vi "PicoScope3000aAWG.vi"(6 "Arbitrary Waveform Settings":T2 {"Index Mode" items=["Single", "Dual", "Quad"]}, 7 "Standard Waveform Settings":T3={"Start Frequency"=1000.0, "Stop Frequency"=1000.0, "Increment"=0.0, "Dwell Time (seconds)"=0.0} {"Stop Frequency" min=0.03 max=1000000.0 format="%#_6p"; "Start Frequency" min=0.03 max=1000000.0 format="%#_6p"}, 8 "Device Info":T1, 9 "General AWG Settings":T4={"Peak-to-Peak Voltage (microvolts)"=2000000, "Offset Voltage (microvolts)"=0, "Wave Type"=0, "Sweep Type"=0, "Shots"=0, "Sweeps"=0, "Trigger Type"=0, "Trigger Source"=0, "Ext. Threshold (ADC count)"=0, "White Noise/PRBS"=0} {"White Noise/PRBS" items=["Normal", "White Noise", "PRBS"]; "Trigger Source" items=["None", "Scope Trigger", "Aux. In", "Ext. In", "Software Trigger"]; "Trigger Type" items=["Rising", "Falling", "Gate High", "Gate Low"]; "Sweep Type" items=["Up", "Down", "Up-Down", "Down-Up"]; "Wave Type" items=["Sine"=0, "Square"=1, "Triangle"=2, "Ramp Up"=3, "Ramp Down"=4, "DC"=8, "Arbitrary"=6]}, 10 "Handle In":i16, 11 "error in":errorcluster) -> (0 "Trigger Source Out":i32, 1 "Arbitrary\nWaveform Graph":i16[](graph), 2 "Handle Out":i16, 3 "error out":errorcluster)   [LabVIEW 2010]
doc: "This VI can be used to control the arbitrary waveform generator. Standard waveforms can be selected or arbitrary waveform can be selected under 'Wave Type'. There are three settings clusters: general settings that apply to both arbitrary and standard waveforms, settings that apply only to standard waveforms and settings that apply only to arbitrary waveforms. It is not necessary to connect all of these clusters if only using arbitrary waveforms or only using standard waveforms are required.\n\nWhen selecting arbitrary waveform, it is necessary to specify a text file containing the wave form. This text file should have a single value on each line in the range -1 to 1. For further information on the settings, see descriptions of ps3000aSetSigGenBuiltIn and ps3000aSetSigGenArbitrary."
uses:
  PS3000a.dll
panel:
  # "Sweep is disabled when 'Increment' or 'Dwell Time' is set to 0, then 'Start frequency' is used"
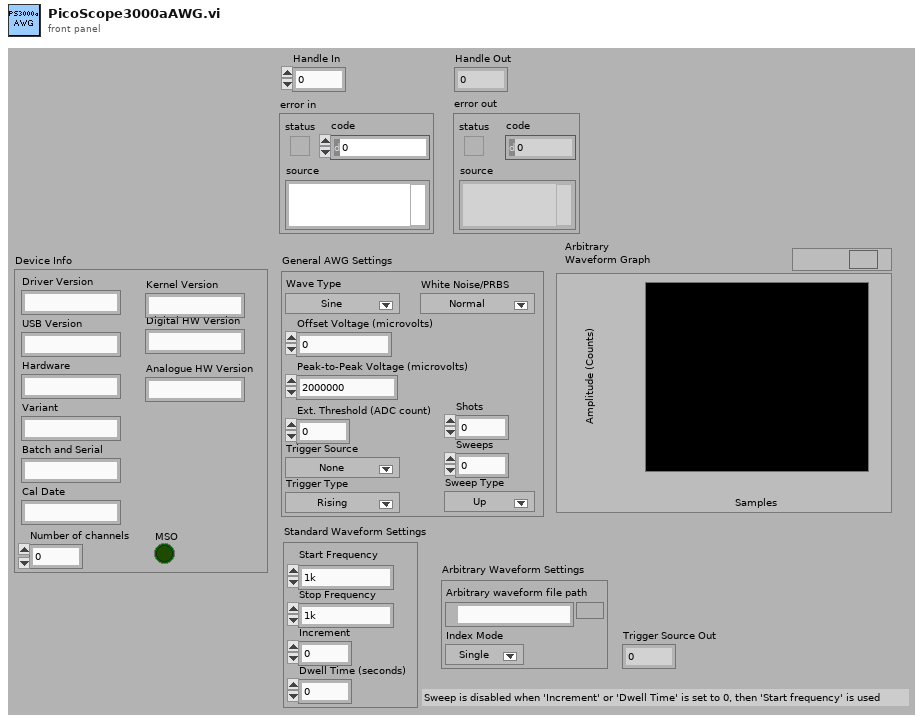
[diagram p1: front panel]
types:
  T1 = cluster{"Driver Version":string, "USB Version":string, "Hardware":string, "Variant":string, "Batch and Serial":string, "Cal Date":string, "Kernel Version":string, "Digital HW Version":string, "Analogue HW Version":string, "MSO":bool, "Number of channels":i16}
  T2 = cluster{"Arbirary waveform file path":path, "Index Mode":u32}
  T3 = cluster{"Start Frequency":dbl, "Stop Frequency":dbl, "Increment":dbl, "Dwell Time (seconds)":dbl}
  T4 = cluster{"Peak-to-Peak Voltage (microvolts)":u32, "Offset Voltage (microvolts)":i32, "Wave Type":i16, "Sweep Type":i32, "Shots":u32, "Sweeps":u32, "Trigger Type":i32, "Trigger Source":i32, "Ext. Threshold (ADC count)":i16, "White Noise/PRBS":u32}
  T5 = cluster{"status":bool, "code":u32, "source":string}
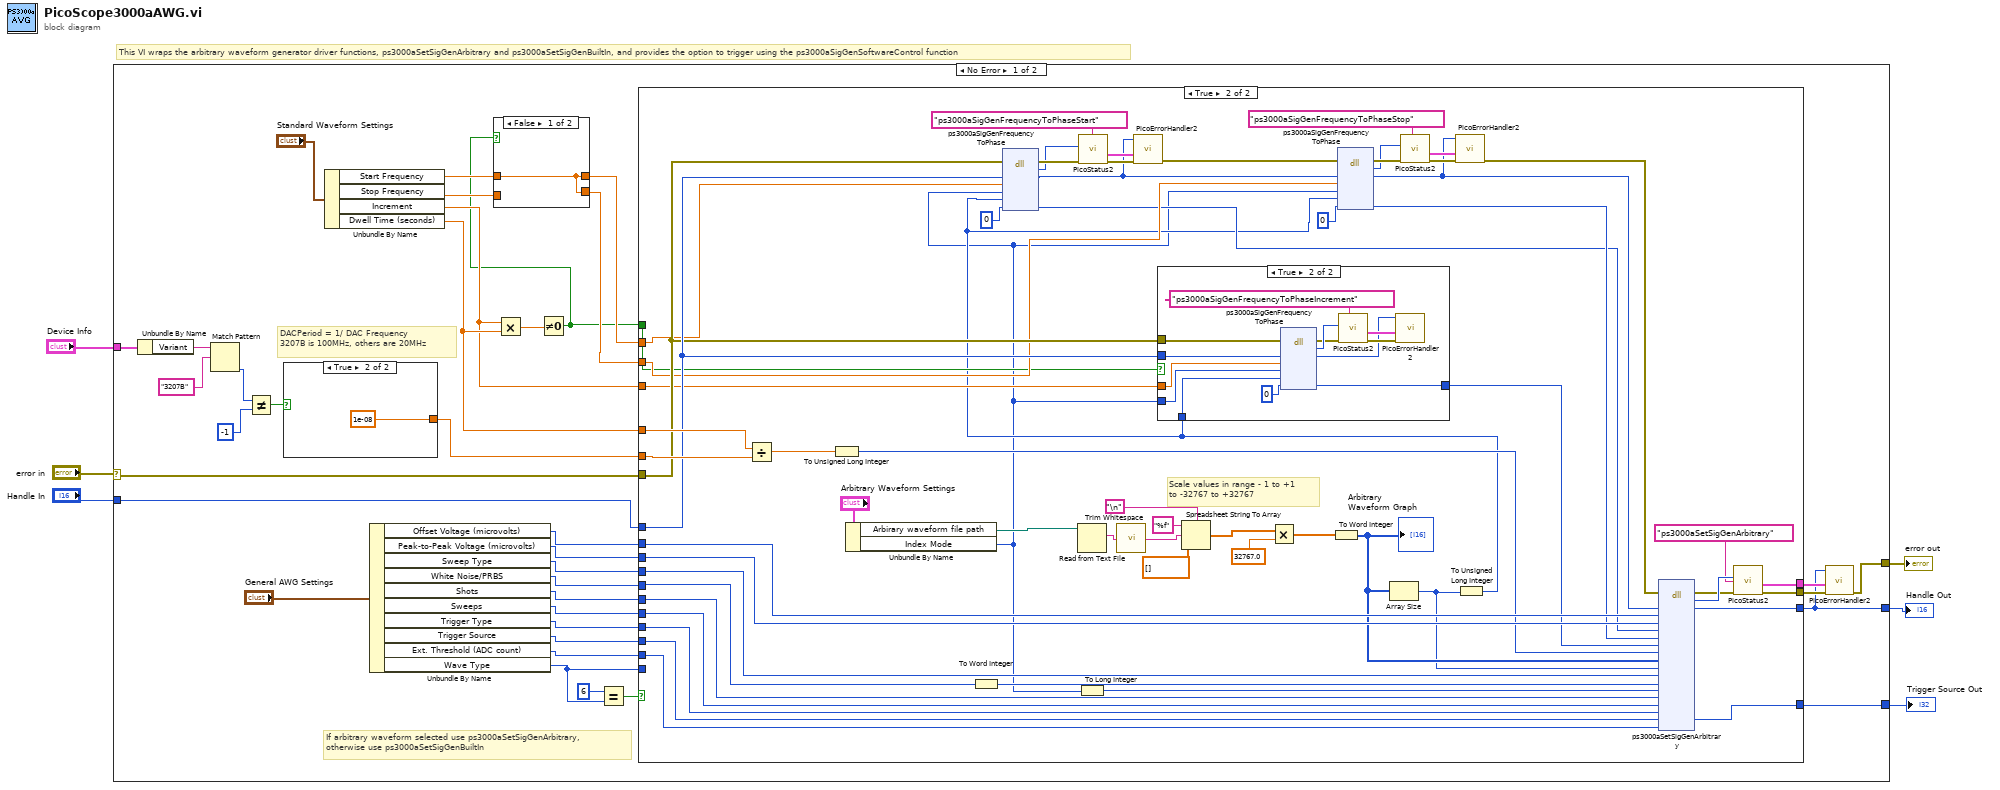
[diagram p0: block diagram]
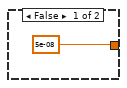
[diagram p2: hidden frame]
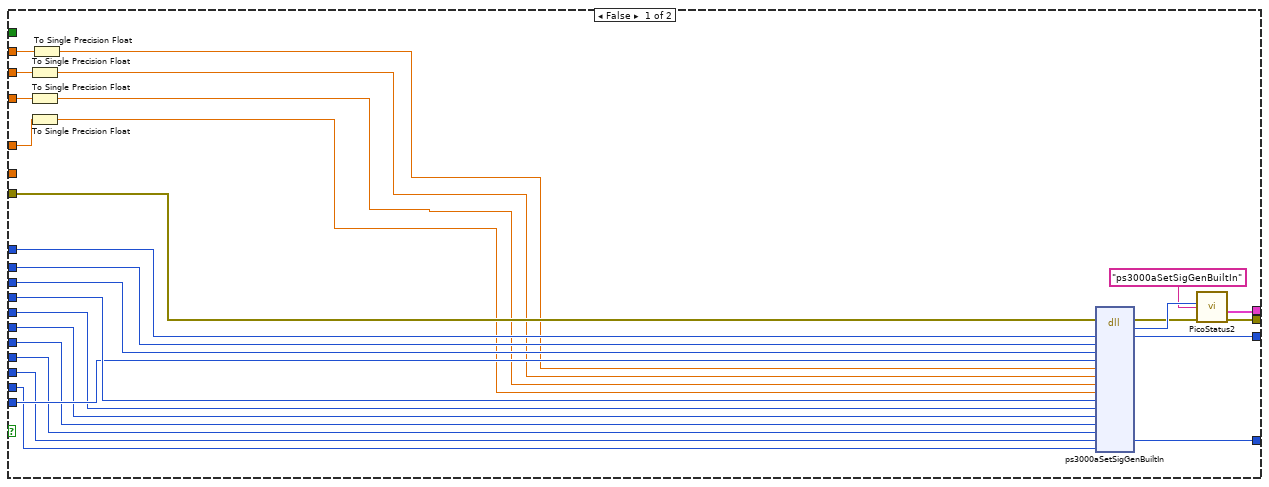
[diagram p4: hidden frame]
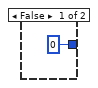
[diagram p5: hidden frame]
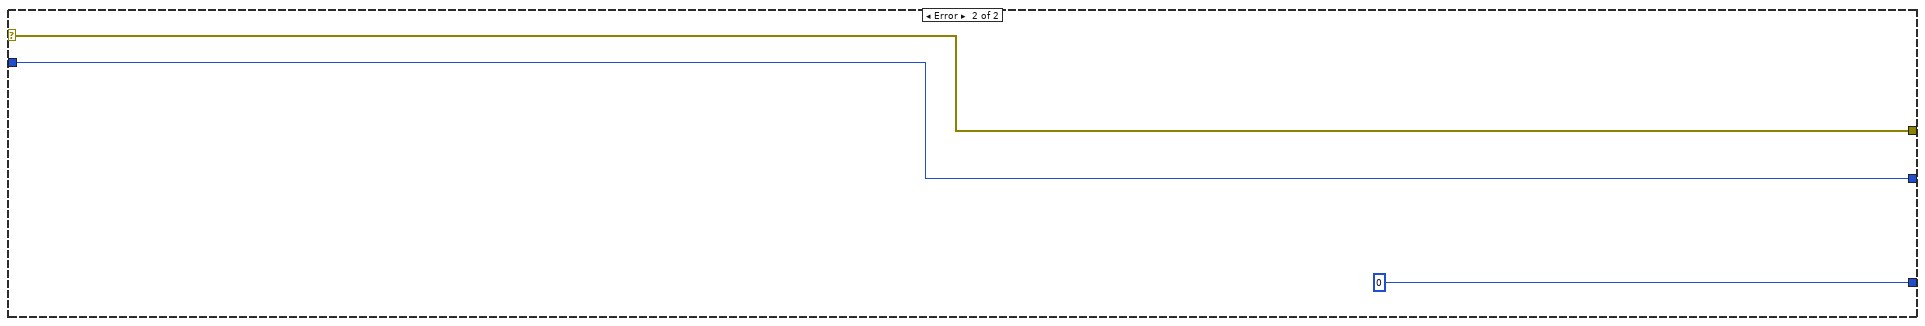
[diagram p6: hidden frame]
diagram:
  # "This VI wraps the arbitrary waveform generator driver functions, ps3000aSetSigGenArbitrary and ps3000aSetSigGenBuiltIn, and provides the option to trigger using the ps3000aSigGenSoftwareControl function"
  n1 = case shown="No Error" "error in" {
    selector: "error in" -> [w27 w152]
    tunnel: [w7 w151] -> w6
    tunnel: "Handle In" -> [w40 w151]
    tunnel: [w39 w152] -> w4
    tunnel: [w25 0] -> w2
    tunnel: "Device Info" -> [w10 _]
    frame No Error {
      # "DACPeriod = 1/ DAC Frequency\n3207B is 100MHz, others are 20MHz"
      # "If arbitrary waveform selected use ps3000aSetSigGenArbitrary, \notherwise use ps3000aSetSigGenBuiltIn"
      n2 = Unbundle By Name(w10) -> ("Variant"=w11:string)
      n3 = Match Pattern(string=w11, regular expression="3207B") -> (offset past match=w12:i32)  [unwired: 1 in, 3 out]
      n4 = Not Equal?(x=w12, y=-1 ("x")) -> (x != y?=w9:bool)
      n5 = case shown="True" w9 {
        tunnel: [5e-08 ("y") 1e-08 ("y")] -> w14
        frame False {
        }
        frame True {
        }
      }
      n6 = Unbundle By Name("Standard Waveform Settings") -> ("Start Frequency"=w23:dbl, "Stop Frequency"=w22:dbl, "Increment"=w19:dbl, "Dwell Time (seconds)"=w20:dbl)
      n7 = Unbundle By Name("General AWG Settings") -> ("Offset Voltage (microvolts)"=w37:i32, "Peak-to-Peak Voltage (microvolts)"=w36:u32, "Sweep Type"=w35:i32, "White Noise/PRBS"=w34:u32, "Shots"=w33:u32, "Sweeps"=w32:u32, "Trigger Type"=w31:i32, "Trigger Source"=w30:i32, "Ext. Threshold (ADC count)"=w29:i16, "Wave Type"=w28:i16)
      n8 = Multiply(x=w19, y=w20) -> (x*y=w21:dbl)
      n9 = Not Equal To 0?(x=w21) -> (x != 0?=w16:bool)
      n10 = case shown="False" w16 {
        tunnel: [w45 w47] -> w18
        tunnel: w22 -> [_ w47]
        tunnel: w23 -> [w45 w46]
        tunnel: [w45 w46] -> w17
        frame False {
        }
        frame True {
        }
      }
      n11 = Equal?(x=i16 6, y=w28) -> (x = y?=w42:bool)
      n12 = case shown="True" w42 {
        tunnel: [w74 w130] -> w7
        tunnel: w40 -> [w73 w96]
        tunnel: [w71 w127] -> w26
        tunnel: w37 -> [w69 w126]
        tunnel: w36 -> [w68 w125]
        tunnel: w35 -> [w67 w124]
        tunnel: w34 -> [w49 w83]
        tunnel: w33 -> [w65 w123]
        tunnel: w32 -> [w64 w122]
        tunnel: w31 -> [w63 w121]
        tunnel: w30 -> [w62 w120]
        tunnel: w29 -> [w61 w119]
        tunnel: w28 -> [w66 _]
        tunnel: [w60 w117] -> w25
        tunnel: w27 -> [w59 w95]
        tunnel: w20 -> [w57 w110]
        tunnel: w19 -> [w56 w92]
        tunnel: w18 -> [w55 w93]
        tunnel: w17 -> [w54 w94]
        tunnel: w14 -> [_ w111]
        tunnel: w16 -> [_ w87]
        tunnel: [w48 w75] -> w8
        frame False {
          n13 = To Single Precision Float(number=w55) -> (single precision float=w51:sgl)
          n14 = To Single Precision Float(number=w56) -> (single precision float=w52:sgl)
          n15 = To Single Precision Float(number=w57) -> (single precision float=w53:sgl)
          n16 = To Single Precision Float(number=w54) -> (single precision float=w50:sgl)
          n17 = dll-call lib="ps3000a.dll" fn="ps3000aSetSigGenBuiltIn" ("ps3000.dll:_ps3000_open_unit@0")(error in=w59, "handle"=w73, "offsetVoltage"=w69, "pkToPk"=w68, "waveType"=w66, "startFrequency"=w50, "stopFrequency"=w51, "increment"=w52, "dwellTime"=w53, "sweepType"=w67, "whiteNoise"=w49, "shots"=w65, "sweeps"=w64, "triggerType"=w63, "triggerSource"=w62, "extInThreshold"=w61) -> (error out=w58:errorcluster, "PICO_STATUS"=w72:u32, "handle"=w74:i16, "triggerSource"=w60:i32)  [unwired: 15 in, 1 out]
          n18 = call "PicoStatus2.vi"("PICO source"="ps3000aSetSigGenBuiltIn" ("source"), "Error in"=w58, "PICO STATUS"=w72) -> ("error out"=w71:errorcluster, "PICO_STATUS out"=w48:T5)  [unwired: 5 in]
        }
        frame True {
          # "Scale values in range - 1 to +1 \nto -32767 to +32767"
          n19 = Divide(x=w110, y=w111) -> (x/y=w112:dbl)
          n20 = To Unsigned Long Integer(number=w112) -> (unsigned 32bit integer=w109:u32)
          n21 = Unbundle By Name("Arbitrary Waveform Settings") -> ("Arbirary waveform file path"=w84:path, "Index Mode"=w80:u32)
          n22 = To Word Integer(number=w83) -> (16bit integer=w82:i16)
          n23 = Read from Text File(file (use dialog)=w84) -> (text=w114:string)  [unwired: 3 in, 3 out]
          n24 = To Long Integer(number=w80) -> (32bit integer=w81:i32)
          n25 = call <vilib>:"Trim Whitespace.vi"("string"=w114) -> ("trimmed string"=w113:string)  [unwired: 1 in]
          n26 = Spreadsheet String To Array(delimiter (Tab)="\n", format string="%f", spreadsheet string=w113, array type (2D Dbl)=dbl[] []) -> (array=w131:dbl[])
          n27 = Multiply(x=w131, y=32767.0 ("deltaPhaseIncrement")) -> (x*y=w115:dbl[])
          n28 = To Word Integer(number=w115) -> (16bit integer=w118:i16[])
          "Arbitrary\nWaveform Graph" <- w118
          n29 = Array Size(array=w118) -> (size(s)=w108:i32)
          n30 = To Unsigned Long Integer(number=w108) -> (unsigned 32bit integer=w86:u32)
          n31 = dll-call lib="ps3000a.dll" fn="ps3000aSigGenFrequencyToPhase" ("ps3000.dll:_ps3000_open_unit@0")(error in=w95, "handle"=w96, "frequency"=w94, "indexMode"=w80, "bufferLength"=w86, "phase"=u32 0) -> (error out=w105:errorcluster, "PICO_STATUS"=w104:u32, "handle"=w78:i16, "phase"=w89:u32)  [unwired: 5 in, 1 out]
          n32 = call "PicoStatus2.vi"("PICO source"="ps3000aSigGenFrequencyToPhaseStart" ("source"), "Error in"=w105, "PICO STATUS"=w104) -> ("error out"=w107:errorcluster, "PICO_STATUS out"=w79:T5)  [unwired: 5 in]
          n33 = call "PicoErrorHandler2.vi"("error in (no error)"=w107, "PICO_STATUS in"=w79, "handle In"=w78) -> ("error out"=w99:errorcluster)  [unwired: 8 in]
          n34 = case shown="True" w87 {
            tunnel: w95 -> [_ w145]
            tunnel: w96 -> [_ w144]
            tunnel: w92 -> [_ w143]
            tunnel: w86 -> [_ w141]
            tunnel: [u32 0 ("phase") w140] -> w88
            tunnel: w80 -> [_ w139]
            frame False {
            }
            frame True {
              n35 = dll-call lib="ps3000a.dll" fn="ps3000aSigGenFrequencyToPhase" ("ps3000.dll:_ps3000_open_unit@0")(error in=w145, "handle"=w144, "frequency"=w143, "indexMode"=w139, "bufferLength"=w141, "phase"=u32 0) -> (error out=w148:errorcluster, "PICO_STATUS"=w149:u32, "handle"=w137:i16, "phase"=w140:u32)  [unwired: 5 in, 1 out]
              n36 = call "PicoStatus2.vi"("PICO source"="ps3000aSigGenFrequencyToPhaseIncrement" ("source"), "Error in"=w148, "PICO STATUS"=w149) -> ("error out"=w146:errorcluster, "PICO_STATUS out"=w138:T5)  [unwired: 5 in]
              n37 = call "PicoErrorHandler2.vi"("error in (no error)"=w146, "PICO_STATUS in"=w138, "handle In"=w137) -> ()  [unwired: 8 in, 1 out]
            }
          }
          n38 = dll-call lib="ps3000a.dll" fn="ps3000aSigGenFrequencyToPhase" ("ps3000.dll:_ps3000_open_unit@0")(error in=w99, "handle"=w78, "frequency"=w93, "indexMode"=w80, "bufferLength"=w86, "phase"=u32 0) -> (error out=w101:errorcluster, "PICO_STATUS"=w100:u32, "handle"=w76:i16, "phase"=w90:u32)  [unwired: 5 in, 1 out]
          n39 = call "PicoStatus2.vi"("PICO source"="ps3000aSigGenFrequencyToPhaseStop" ("source"), "Error in"=w101, "PICO STATUS"=w100) -> ("error out"=w103:errorcluster, "PICO_STATUS out"=w77:T5)  [unwired: 5 in]
          n40 = call "PicoErrorHandler2.vi"("error in (no error)"=w103, "PICO_STATUS in"=w77, "handle In"=w76) -> ("error out"=w91:errorcluster)  [unwired: 8 in]
          n41 = dll-call lib="ps3000a.dll" fn="ps3000aSetSigGenArbitrary" ("ps3000.dll:_ps3000_open_unit@0")(error in=w91, "handle"=w76, "offsetVoltage"=w126, "pkToPk"=w125, "startDeltaPhase"=w89, "stopDeltaPhase"=w90, "deltaPhaseIncrement"=w88, "dwellCount"=w109, "arbitraryWaveform"=w118, "arbitraryWaveformSize"=w108, "sweepType"=w124, "whiteNoise"=w82, "indexMode"=w81, "shots"=w123, "sweeps"=w122, "triggerType"=w121, "triggerSource"=w120, "extInThreshold"=w119) -> (error out=w116:errorcluster, "PICO_STATUS"=w129:u32, "handle"=w130:i16, "triggerSource"=w117:i32)  [unwired: 17 in, 1 out]
          n42 = call "PicoStatus2.vi"("PICO source"="ps3000aSetSigGenArbitrary" ("source"), "Error in"=w116, "PICO STATUS"=w129) -> ("error out"=w127:errorcluster, "PICO_STATUS out"=w75:T5)  [unwired: 5 in]
        }
      }
      n43 = call "PicoErrorHandler2.vi"("error in (no error)"=w26, "PICO_STATUS in"=w8, "handle In"=w7) -> ("error out"=w39:errorcluster)  [unwired: 8 in]
    }
    frame Error {
    }
  }
  "Handle Out" <- w6
  "error out" <- w4
  "Trigger Source Out" <- w2
